vi "RFmxSpecAn Get Results(Harms).vi"(0 "SA Handle In":refnum<k21> caption="Instrument Handle In", 2 "# of Harms":i32=1 min=1 max=10, 3 "STOP":refnum<vi>, 5 "SG Handle In":refnum<k15>, 11 "error in (no error)":errorcluster, 12 "Spectrum":refnum<vi>, 13 "Marker Level":refnum<vi>, 14 "Marker Freq":refnum<vi>) -> (4 "SA Handle Out":refnum<k21> caption="Instrument Handle Out", 6 "SG handle out":refnum<k15>, 15 "error out":errorcluster)   [LabVIEW 2018]
panel:
  out "Freq":dbl
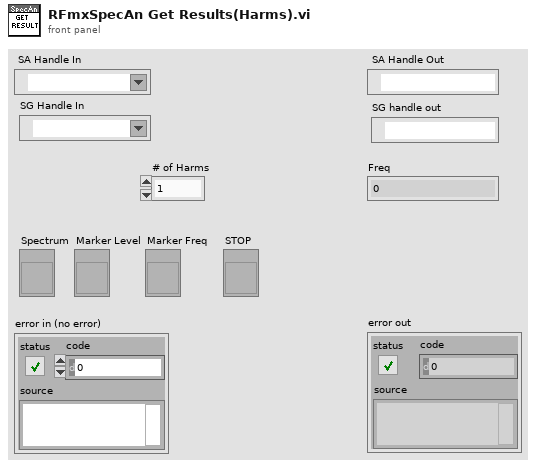
[diagram p1: front panel]
types:
  T1 = typedef "niRFmx Instrument Handle.ctl" = refnum<k21>
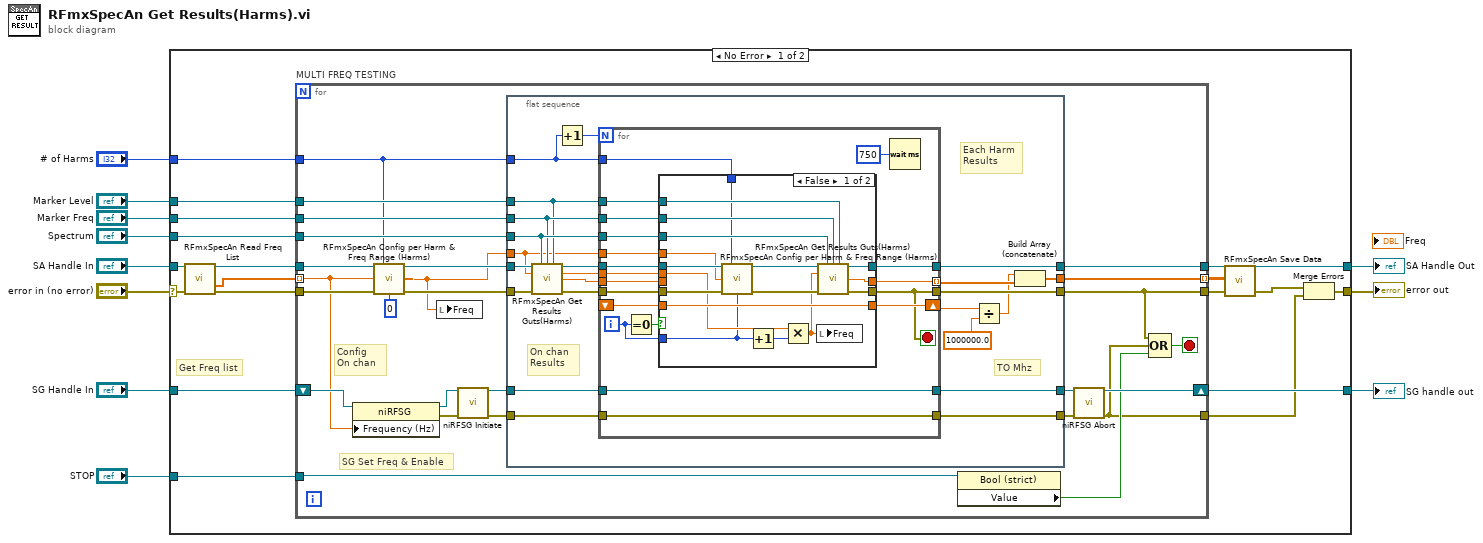
[diagram p0: block diagram]
diagram:
  n1 = case shown="No Error" "error in (no error)" {
    selector: "error in (no error)" -> [w22 w119]
    tunnel: "SA Handle In" -> [w28 w120]
    tunnel: [w16 w119] -> w9
    tunnel: [w19 w120] -> w8
    tunnel: "Spectrum" -> [w27 _]
    tunnel: "Marker Level" -> [w25 _]
    tunnel: "Marker Freq" -> [w26 _]
    tunnel: "SG Handle In" -> [w23 w118]
    tunnel: [w21 w118] -> w3
    tunnel: "# of Harms" -> [w13 _]
    tunnel: "STOP" -> [w12 _]
    frame No Error {
      # "Get Freq list"
      n2 = call "RFmxSpecAn Read Freq List.vi"("error in (no error)"=w22) -> ("Freq List (Hz)"=w14:dbl[], "error out"=w24:errorcluster)  [unwired: 13 in]
      n3 = for "MULTI FREQ TESTING" {
        tunnel: w28 -> [w40]
        tunnel: w27 -> [w54]
        tunnel: w26 -> [w53]
        tunnel: w25 -> [w52]
        tunnel: [w47] -> w19
        tunnel: [w30] -> w17
        tunnel: w13 -> [w36]
        tunnel: [w42] -> w15 mode=indexing
        shift-right: [w50] -> w21
        shift-left: w23 -> [w51]
        tunnel: w14 -> [w37] mode=indexing
        tunnel: w24 -> [w39]
        tunnel: [w33] -> w20
        tunnel: w12 -> [w32]
        stop <- w34 stop-if-true
        # "Config \nOn chan"
        # "SG Set Freq & Enable"
        n4 = property class="niRFSG"(reference=w51, "Frequency (Hz)"=w37) -> (reference out=w48:refnum<k15>, error out=w49:errorcluster)  [unwired: 1 in]
        n5 = call "RFmxSpecAn Config per Harm & Freq Range (Harms).vi"("SA Handle In"=w40, "# of Harms"=w36, "Center Freq (Hz) In"=w37, "error in (no error)"=w39, "Meas Harm #"=u8 0) -> ("SA Handle Out"=w41:refnum<k21>, "Center Freq (Hz) Out"=w29:dbl, "error out"=w38:errorcluster)  [unwired: 8 in]
        n6 = local write "Freq"(w29) -> ()
        n7 = call <instrlib>:"niRFSG Initiate.vi"("instrument handle"=w48, "error in"=w49) -> ("instrument handle out"=w45:refnum<k15>, "error out"=w46:errorcluster)  [unwired: 12 in]
        n8 = flat-sequence {
          tunnel: w41 -> [w69]
          tunnel: w54 -> [w65]
          tunnel: w53 -> [w64]
          tunnel: w52 -> [w63]
          tunnel: w38 -> [w68]
          tunnel: [w77] -> w33
          tunnel: [w76] -> w47
          tunnel: w46 -> [w75]
          tunnel: w45 -> [w74]
          tunnel: [w73] -> w44
          tunnel: [w72] -> w43
          tunnel: w36 -> [w56]
          tunnel: [w61] -> w42
          tunnel: w29 -> [w55]
          frame #0 {
            # "TO Mhz"
            # "Each Harm\nResults"
            # "On chan \nResults"
            n9 = call "RFmxSpecAn Get Results Guts(Harms).vi"("Refnum in"=w69, "Spectrum in"=w65, "Marker Freq"=w64, "Marker Level"=w63, "Center Freq (Hz)"=w55, "error in (no error)"=w68) -> ("Refnum out"=w66:T1, "Peak Frequency (Hz)"=w71:dbl, "Peak Amplitude"=w70:dbl, "error out"=w67:errorcluster)  [unwired: 6 in]
            n10 = Increment(x=w56) -> (x+1=w57:i32)
            n11 = for {
              N: w57 -> [_]
              tunnel: w66 -> [w96]
              tunnel: w65 -> [w95]
              tunnel: w64 -> [w94]
              tunnel: w63 -> [w93]
              tunnel: w67 -> [w92]
              tunnel: [w80] -> w77
              tunnel: [w91] -> w76
              tunnel: w75 -> [w90]
              tunnel: w74 -> [w89]
              tunnel: [w90] -> w72
              tunnel: [w89] -> w73
              tunnel: w71 -> [w87]
              tunnel: w70 -> [w86]
              shift-right: [w84] -> w60
              shift-left: _ -> [w83]
              tunnel: [w82] -> w62 mode=indexing
              tunnel: w56 -> [w81]
              tunnel: w55 -> [w78]
              i -> [w79]
              stop <- w80 stop-if-true
              n12 = Equal To 0?(x=w79) -> (x = 0?=w85:bool)
              n13 = case shown="False" w85 {
                tunnel: w96 -> [w104 w116]
                tunnel: w95 -> [w113 _]
                tunnel: w94 -> [w112 _]
                tunnel: w93 -> [w111 _]
                tunnel: w92 -> [w106 w117]
                tunnel: [w110 w117] -> w80
                tunnel: [w109 w116] -> w91
                tunnel: w87 -> [w99 w114]
                tunnel: w86 -> [_ w115]
                tunnel: [w108 w114] -> w84
                tunnel: w83 -> [w108 _]
                tunnel: [w107 w115] -> w82
                tunnel: w81 -> [w102 _]
                tunnel: w79 -> [w97 _]
                tunnel: w78 -> [w100 _]
                frame False {
                  n14 = call "RFmxSpecAn Config per Harm & Freq Range (Harms).vi"("SA Handle In"=w104, "# of Harms"=w102, "Center Freq (Hz) In"=w100, "error in (no error)"=w106, "Meas Harm #"=w97) -> ("SA Handle Out"=w103:refnum<k21>, "error out"=w105:errorcluster)  [unwired: 8 in, 1 out]
                  n15 = Increment(x=w97) -> (x+1=w98:i32)
                  n16 = Multiply(x=w99, y=w98) -> (x*y=w101:dbl)
                  n17 = local write "Freq"(w101) -> ()
                  n18 = call "RFmxSpecAn Get Results Guts(Harms).vi"("Refnum in"=w103, "Spectrum in"=w113, "Marker Freq"=w112, "Marker Level"=w111, "Center Freq (Hz)"=w101, "error in (no error)"=w105) -> ("Refnum out"=w109:T1, "Peak Amplitude"=w107:dbl, "error out"=w110:errorcluster)  [unwired: 6 in, 1 out]
                }
                frame True {
                }
              }
              n19 = Wait (ms)(milliseconds to wait=u32 750) -> ()  [unwired: 1 out]
            }
            n20 = Divide(x=w60, y=1000000.0) -> (x/y=w59:dbl)
            n21 = Build Array (concatenate)(w59, w62) -> (w61:dbl[])
          }
        }
        n22 = property class="Bool (strict)"(reference=w32) -> ("Value"=w31:bool)  [unwired: 1 in, 2 out]
        n23 = call <instrlib>:"niRFSG Abort.vi"("instrument handle"=w44, "error in"=w43) -> ("instrument handle out"=w50:refnum<k15>, "error out"=w30:errorcluster)  [unwired: 12 in]
        n24 = Compound Arithmetic op=OR(w33, w30, w31) -> (w34:bool)
      }
      n25 = call "RFmxSpecAn Save Data.vi"("error in (no error)"=w20, "Harms Results"=w15) -> ("error out"=w18:errorcluster)  [unwired: 3 in]
      n26 = Merge Errors(w18, w17) -> (w16:errorcluster)
    }
    frame Error {
    }
  }
  "error out" <- w9
  "SA Handle Out" <- w8
  "SG handle out" <- w3
